vi "Global 1.vi"() -> ()   [LabVIEW 2014]
panel:
  in  "Lift Inhibit":bool
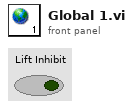
[diagram p1: front panel]
diagram:
